vi "Sep_Bool.vi"(2 "output cluster":T2, 3 "Relay_Channel_Write":T3) -> (0 "DO_Bool":bool[](array[boolean]), 1 "Array":T1[](array[typedef]))   [LabVIEW 2024, in "Relay_Module.lvlib"]
uses:
  Relay_Module.lvlib
  Relay_Channel_Write.ctl
  Relay_Enum_OUT.ctl
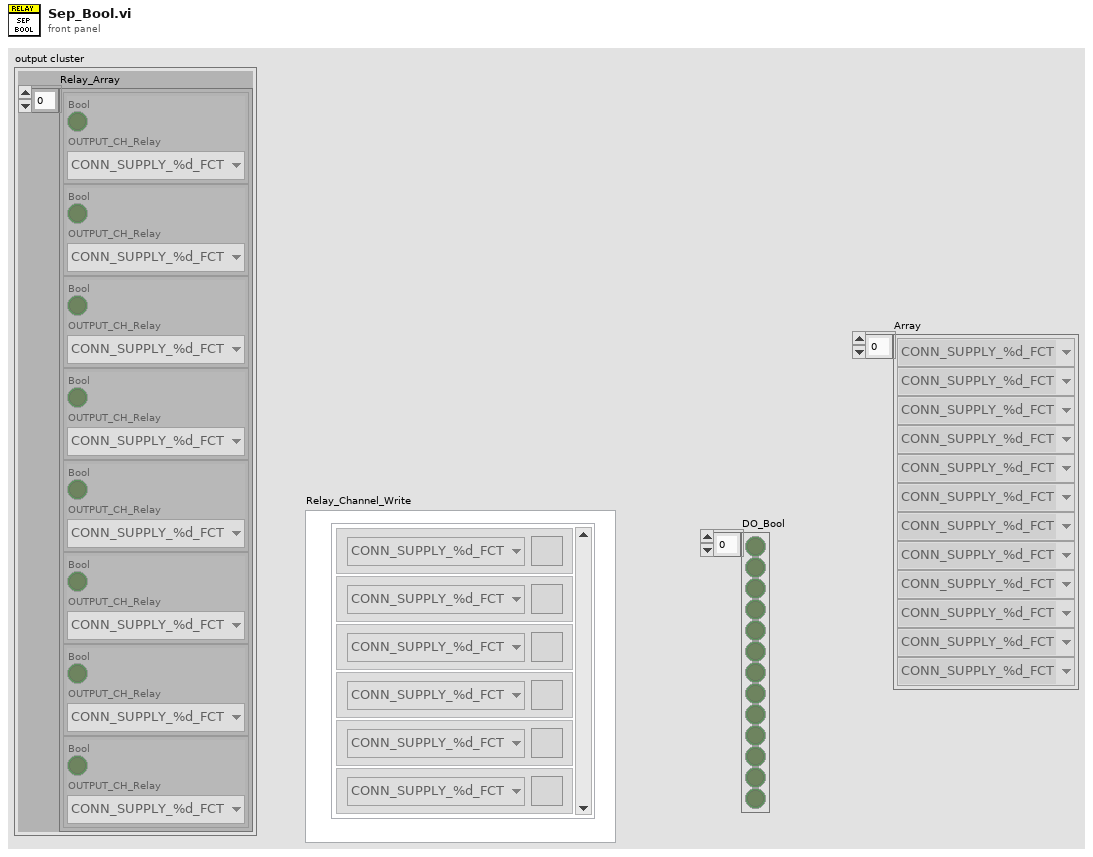
[diagram p1: front panel]
types:
  T1 = typedef "Relay_Module.lvlib/Relay_Enum_OUT.ctl" = enum16{"CONN_SUPPLY_%d_FCT", "HB_CONN_%d_FCT", "L_IND_CONN_%d_FCT", "R_IND_CONN_%d_FCT", "SW1_%d_FCT", "SW2_%d_FCT", "CAN_H_%d_FCT", "CAN_L_%d_FCT", "CYLINDER_ON/OFF_%d_FCT", "SPARE_1_%d_FCT", "SPARE_2_%d_FCT", "Tower Red", "Tower Amber", "Tower Green", "Tower Buzzer", "SLIMRELAY_DUT_%d_FCT", "GND_DMM_%d_EOL", "CAN_H_RES_%d_EOL", "CAN_L_RES_%d_EOL", "L_IND_RES_%d_EOL", "R_IND_RES_%d_EOL", "HB_CONN_DMM_%d_EOL", "14V_RES_%d_EOL", "CAN_L_(DMM-)_%d_EOL", "CAN_H_%d_EOL", "CAN_L_%d_EOL", "14V_%d_EOL", "GND_%d_EOL", "HB_CONN_%d_EOL", "L_IND_%d_EOL", "R_IND_%d_EOL", "CYLINDER_DUT_%d_EOL", "CYL_PB_1_%d_EOL", "CYL_PB_2_%d_EOL", "DUT_PASS_%d_EOL", "DUT_FAIL_%d_EOL", "SPARE1_%d_EOL", "Tower Red_EOL", "Tower Amber_EOL", "Tower Green_EOL", "Tower Buzzer_EOL"}
  T2 = cluster{"Relay_Array":cluster{"Bool":bool, "OUTPUT_CH_Relay":T1}[]}
  T3 = typedef "Relay_Module.lvlib/Relay_Channel_Write.ctl" = cluster{"Relay_CH_Array":cluster{"On/Off":bool, "OUTPUT_Relay_Channels":T1}[]}
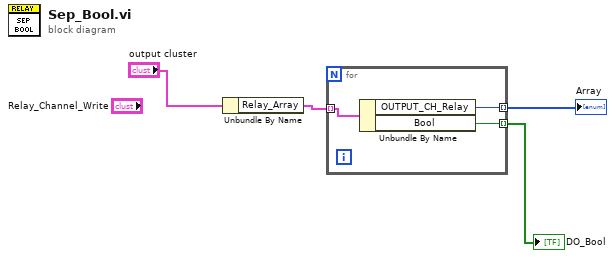
[diagram p0: block diagram]
diagram:
  n1 = Unbundle By Name("output cluster") -> ("Relay_Array"=w4:cluster{"Bool":bool, "OUTPUT_CH_Relay":T1}[])
  n2 = for {
    tunnel: w4 -> [w7] mode=indexing
    tunnel: [w6] -> w2 mode=indexing
    tunnel: [w5] -> w3 mode=indexing
    n3 = Unbundle By Name(w7) -> ("OUTPUT_CH_Relay"=w6:T1, "Bool"=w5:bool)
  }
  "DO_Bool" <- w3
  "Array" <- w2
